vi "LaunchPad Command Loop.vi"   [LabVIEW 2015]
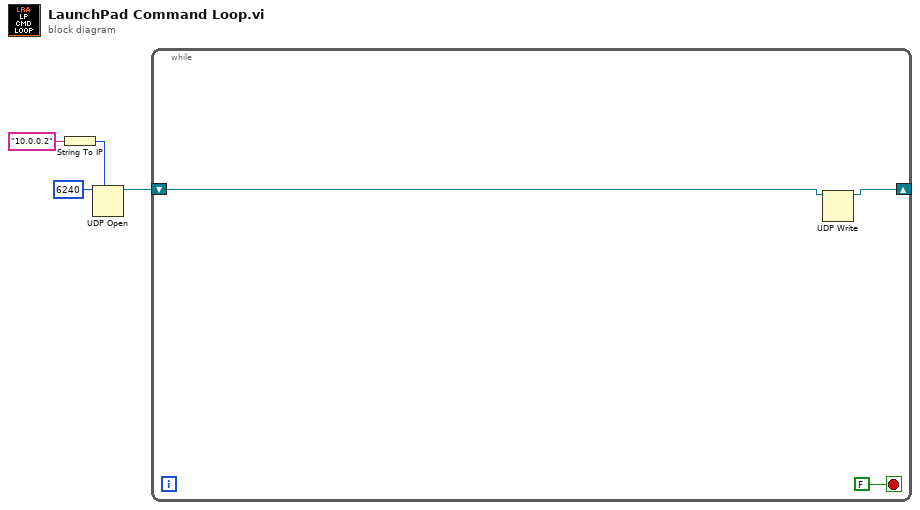
[diagram p0: block diagram]
diagram:
  n1 = String To IP(1:"10.0.0.2" ("name")) -> (0:w4:u32)
  n2 = UDP Open(7:w4, 11:u16 6240 ("port")) -> (port=w1:refnum<k16>)  [unwired: 3 in, 2 out]
  n3 = while {
    shift-right: [w5] -> _
    shift-left: w1 -> [w6]
    stop <- FALSE stop-if-true
    n4 = UDP Write(connection ID=w6) -> (3:w5:refnum<k16>)  [unwired: 5 in, 1 out]
  }
